vi "mod_LDPC Calculate Likelihoods.vi"   [LabVIEW 2020, in "niDMT.lvlib"]
uses:
  <vilib>/addons/Modulation/niDMT.lvlib
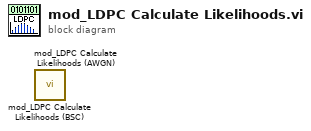
[diagram p0: block diagram]
diagram:
  n1 = call <vilib>:"mod_LDPC Calculate Likelihoods (BSC).vi"() -> ()  [unwired: 14 in, 2 out]
  n2 = call <vilib>:"mod_LDPC Calculate Likelihoods (AWGN).vi"() -> ()  [unwired: 14 in, 2 out]
